vi "Read key-value pairs.vi"(8 "error in":errorcluster, 11 "CEF_serializable configuration in":refnum<class "CEF_serializable configuration.lvclass">) -> (0 "error out":errorcluster, 2 "key-value pairs":string[][](array[string]), 3 "CEF_serializable configuration out":refnum<class "CEF_serializable configuration.lvclass">)   [LabVIEW 2025, in "CEF.lvlib" / "CEF_serializable configuration.lvclass"]
doc: "Copyright 2017 National Instruments Corporation\n\nLicensed under the Apache License, Version 2.0 (the \"License\"); you may not use this file except in compliance with the License. You may obtain a copy of the License at http://www.apache.org/licenses/LICENSE-2.0\nUnless required by applicable law or agreed to in writing, software distributed under the License is distributed on an \"AS IS\" BASIS, WITHOUT WARRANTIES OR CONDITIONS OF ANY KIND, either express or implied. See the License for the specific language governing permissions and limitations under the License."
uses:
  CEF_serializable configuration.lvclass
  CEF_serializable configuration.lvclass/CEF_serializable configuration.ctl
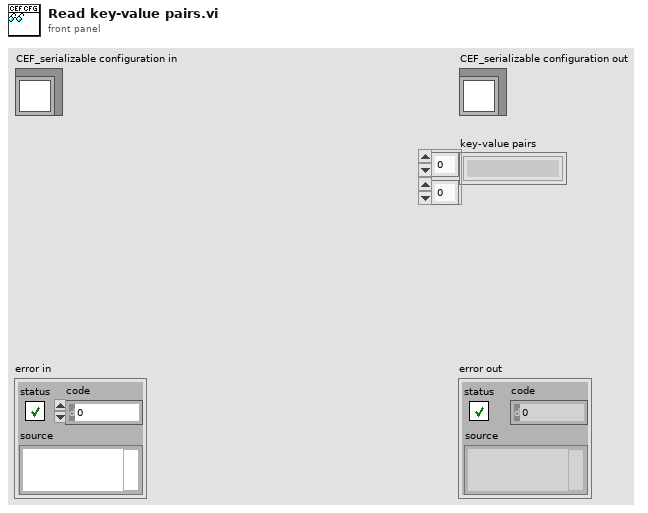
[diagram p1: front panel]
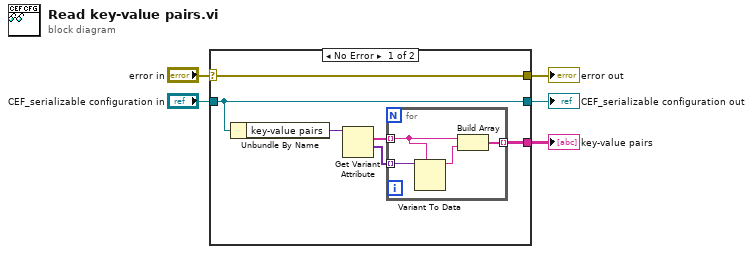
[diagram p0: block diagram]
diagram:
  n1 = case shown="No Error" "error in" {
    selector: "error in" -> [w11 w16]
    tunnel: [w11 w16] -> w4
    tunnel: [w10 w17] -> w2
    tunnel: "CEF_serializable configuration in" -> [w10 w17]
    tunnel: [w6 _] -> w1
    frame No Error {
      n2 = Unbundle By Name(w10) -> ("key-value pairs"=w9:variant)
      n3 = Get Variant Attribute(Variant=w9) -> (names=w8:string[], values=w7:variant[])  [unwired: 3 in, 2 out]
      n4 = for {
        tunnel: w8 -> [w15] mode=indexing
        tunnel: [w13] -> w6 mode=indexing
        tunnel: w7 -> [w12] mode=indexing
        n5 = Variant To Data(type=w15, Variant=w12) -> (data=w14:string)  [unwired: 1 in, 1 out]
        n6 = Build Array(w15, w14) -> (w13:string[])
      }
    }
    frame Error {
    }
  }
  "error out" <- w4
  "CEF_serializable configuration out" <- w2
  "key-value pairs" <- w1
